vi "未公开控件.vi"() -> ()   [LabVIEW 2012]
panel:
  out "颜色梯度":dbl(ramp)
  in  "下拉列表 3":dbl(ring)
  in  "?":u16(ring) items=["AAAA", "BBB"]
  in  "垂直滚动条":i32(c297)
  in  "下拉列表 2":i16(ring)
  in  "下拉列表":u16(ring) items=["Item"]
  in  "滚动条":i32(c297)
  in  "布尔":bool
  in  "多段管道":bool(c317)
  in  "字符串":string
  in  "滑动杆":dbl(slide) scale=0.0..10.0
  in  "数值":dbl
  in  "垂直滑动杆":dbl(slide) scale=0.0..10.0
  out "液罐 7":dbl(slide) scale=0.0..100.0
  out "液罐 6":dbl(slide) scale=0.0..100.0
  out "液罐 5":dbl(slide) scale=0.0..100.0
  out "液罐 4":dbl(slide) scale=0.0..100.0
  out "液罐 3":dbl(slide) scale=0.0..100.0
  out "液罐 2":dbl(slide) scale=0.0..100.0
  out "液罐":dbl(slide) scale=0.0..100.0
  out "漏斗 2":dbl(slide) scale=0.0..100.0
  out "漏斗":dbl(slide) scale=0.0..100.0
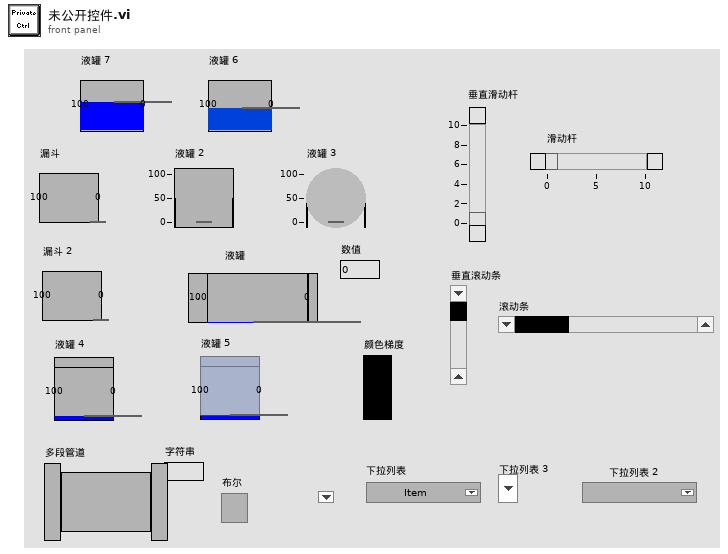
[diagram p1: front panel]
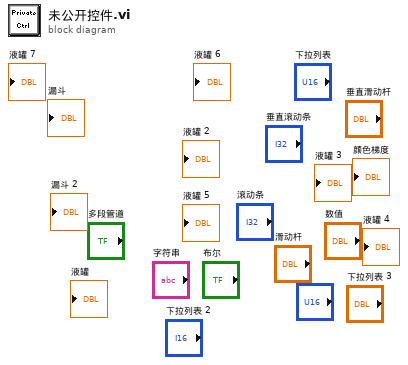
[diagram p0: block diagram]
diagram:
